vi "GlobalValue.vi"() -> ()   [LabVIEW 2013]
uses:
  Controls/DAQConfig.ctl
  SystemCode/SysControl/Setup.ctl
panel:
  out "Slot2USBCOM DY":refnum<visa-resource-name>
  out "Slot1USBCOM DY":refnum<visa-resource-name>
  out "WIFIPW":string
  out "WIFINAME":string
  out "devid":string
  out "CCID info":string[][](array[string])
  out "debug":bool
  out "Slot2QCCOM":refnum<visa-resource-name>
  out "Slot1QCCOM":refnum<visa-resource-name>
  out "SN Result":bool
  out "Slot2-CCID信息":string[](array[string])
  out "Slot1-CCID信息":string[](array[string])
  out "Slot2CCID":string
  out "Slot1CCID":string
  out "Slot2-SIM信息":string[](array[string])
  out "Slot1-SIM信息":string[](array[string])
  in  "MEID-ESN":string[][](array[string])=[["8986031490021881534", "460036161669975", "2A645416CB435F94", "8006A127", "460036161669975@mycdma.cn", "DB60264368A1D188", "18101891253", "A1000021A59070"], ["8986031490021881535", "460036161669976", "32FA5764D69C76BE", "80FAE4E6", "460036161669976@mycdma.cn", "B3AA1B3D2F0D5593", "18964872399", "A1000021A58D61"], ["8986031491021061568", "460036161669995", "AB0626182B92834D", "807395B1", "460036161669995@mycdma.cn", "20BF73A9D3FA03F7", "", "A1000021A635CD"], ["", "", "", "", "", "", "", ""], ["", "", "", "", "", "", "", ""], ["", "", "", "", "", "", "", ""], ["", "", "", "", "", "", "", ""], ["", "", "", "", "", "", "", ""], ["", "", "", "", "", "", "", ""], ["", "", "", "", "", "", "", ""], ["", "各位，模块烧号主要是写五码，包括IMSI、AKEY、MEID（ESN）、AN(EVDO USER)、AAA(EVDO PWD)。", "", "", "", "", "", ""], ["", "其中ESN和MEID在模块出厂时已经写入，两者均可通过AT指令读取，但ESN不可更改。", "", "", "", "", "", ""], ["", "经询问及实际测试，上海电信绑定ESN号而广东电信未绑定，意味着上海电信五码烧录到其它模块是不可用的，但广东电信则无此限制。", "", "", "", "", "", ""], ["", "", "", "", "", "", "", ""], ["", "", "", "", "", "", "", ""], ["", "目前已确定跟上海电信合作，后续模块及卡号使用过程中，如遇到模块损坏，则意味着该卡必须销号（除非向电信申请绑定新的ESN），否则烧录到其它模块中是没用的。", "", "", "", "", "", ""]]
  out "Slot2ESN":string
  out "Slot1ESN":string
  out "Slot2MEID":string
  out "Slot1MEID":string
  in  "Data":string[][](array[string])=[["8986031490021881534", "460036161669975", "2A645416CB435F94", "8006A127", "460036161669975@mycdma.cn", "DB60264368A1D188", "18101891253", "A1000021A59070"], ["8986031490021881535", "460036161669976", "32FA5764D69C76BE", "80FAE4E6", "460036161669976@mycdma.cn", "B3AA1B3D2F0D5593", "18964872399", "A1000021A58D61"], ["8986031491021061568", "460036161669995", "AB0626182B92834D", "807395B1", "460036161669995@mycdma.cn", "20BF73A9D3FA03F7", "", "A1000021A635CD"], ["", "", "", "", "", "", "", ""], ["", "", "", "", "", "", "", ""], ["", "", "", "", "", "", "", ""], ["", "", "", "", "", "", "", ""], ["", "", "", "", "", "", "", ""], ["", "", "", "", "", "", "", ""], ["", "", "", "", "", "", "", ""], ["", "各位，模块烧号主要是写五码，包括IMSI、AKEY、MEID（ESN）、AN(EVDO USER)、AAA(EVDO PWD)。", "", "", "", "", "", ""], ["", "其中ESN和MEID在模块出厂时已经写入，两者均可通过AT指令读取，但ESN不可更改。", "", "", "", "", "", ""], ["", "经询问及实际测试，上海电信绑定ESN号而广东电信未绑定，意味着上海电信五码烧录到其它模块是不可用的，但广东电信则无此限制。", "", "", "", "", "", ""], ["", "", "", "", "", "", "", ""], ["", "", "", "", "", "", "", ""], ["", "目前已确定跟上海电信合作，后续模块及卡号使用过程中，如遇到模块损坏，则意味着该卡必须销号（除非向电信申请绑定新的ESN），否则烧录到其它模块中是没用的。", "", "", "", "", "", ""]]
  out "Slot2USB":string
  out "Slot1USB":string
  out "Slot2USBCOM":refnum<visa-resource-name>
  out "Slot1USBCOM":refnum<visa-resource-name>
  out "Slot2COM":refnum<visa-resource-name>
  out "Slot1COM":refnum<visa-resource-name>
  out "MainViPath":path
  out "ConfigOut":T1={"TestedNum"=10, "PassedNum"=5, "FailedNum"=5, "Slot1TestedNum"=10, "Slot2TestedNum"=10, "Slot3TestedNum"=10, "Slot4TestedNum"=10, "GuiVer"="1.0", "LimitFileVer"="1.0", "Login Name"="", "Password"="", "SN_Head"="0", "SN_Length"=1, "AbortOnFail"=FALSE, "DataBaseEnable?"=FALSE, "FixtureID"="", "ShowSkipStep?"=FALSE}
  in  "测试项目":string[][](table)
  out "SIMCOM通信协议":string[][](array[string])
  out "通信协议":string[][](array[string])
  out "Instruments":T2(array[cluster])
  out "DAQConfig":T3={"DIO"=[["钥匙keyin", "Dev2/port0/line0", "H", "DI"], ["遥控解锁", "Dev2/port0/line1", "H", "DI"], ["后背门", "Dev2/port0/line2", "H", "DI"], ["车门1", "Dev2/port0/line3", "H", "DI"]], "AO"=[["钥匙keyin", "Dev2/port0/line0", "H", "DI"], ["遥控解锁", "Dev2/port0/line1", "H", "DI"], ["后背门", "Dev2/port0/line2", "H", "DI"], ["车门1", "Dev2/port0/line3", "H", "DI"]], "AI"=[["钥匙keyin", "Dev2/port0/line0", "H", "DI"], ["遥控解锁", "Dev2/port0/line1", "H", "DI"], ["后背门", "Dev2/port0/line2", "H", "DI"], ["车门1", "Dev2/port0/line3", "H", "DI"]]}
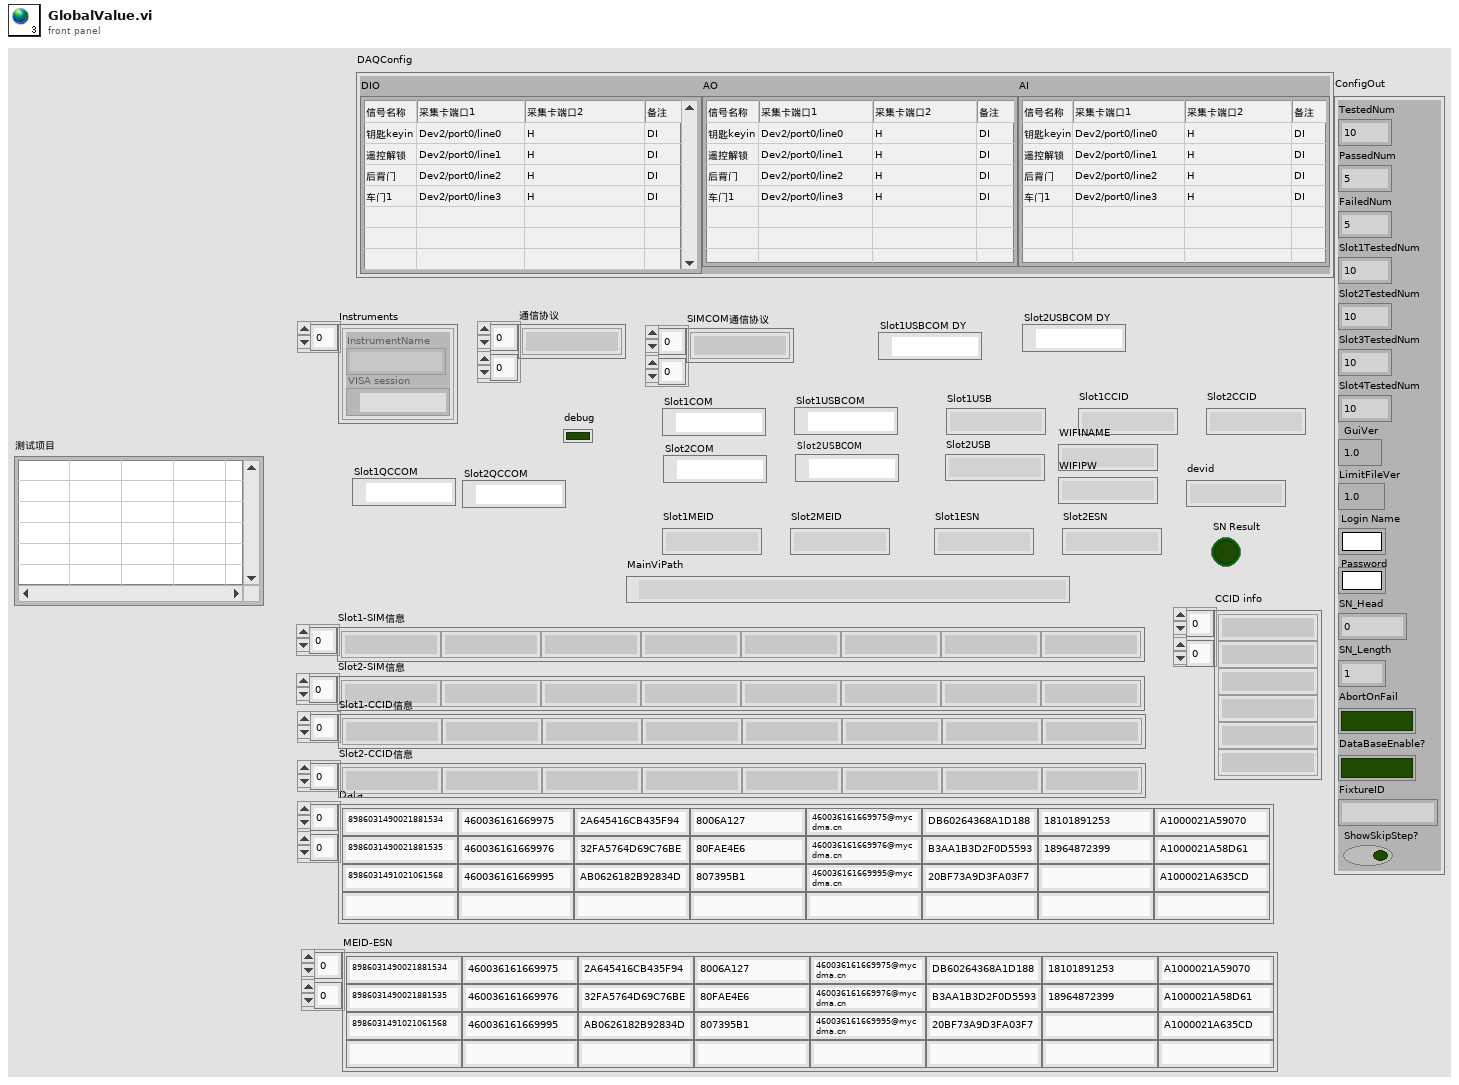
[diagram p1: front panel]
types:
  T1 = typedef "Setup.ctl" = cluster{"TestedNum":u32, "PassedNum":u32, "FailedNum":u32, "Slot1TestedNum":u32, "Slot2TestedNum":u32, "Slot3TestedNum":u32, "Slot4TestedNum":u32, "GuiVer":string, "LimitFileVer":string, "Login Name":string, "Password":string, "SN_Head":string, "SN_Length":i32, "AbortOnFail":bool, "DataBaseEnable?":bool, "FixtureID":string, "ShowSkipStep?":bool}
  T2 = cluster{"InstrumentName":string, "VISA session":refnum<visa-resource-name>}[]
  T3 = typedef "DAQConfig.ctl" = cluster{"DIO":string[][], "AO":string[][], "AI":string[][]}
diagram:
